vi "Arrange_FrontPanel_Object.vi"(0 "vi refnum":refnum<vi>, 7 "spacing":i32=15, 11 "error in (no error)":errorcluster) -> (4 "vi refnum out":refnum<vi>, 15 "error out":errorcluster)   [LabVIEW 2017]
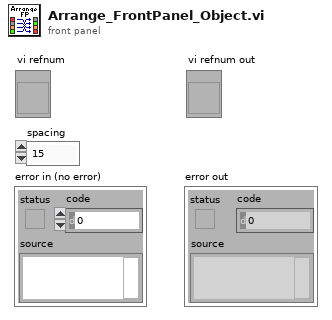
[diagram p1: front panel]
types:
  T1 = cluster{"Ctl Refnum":refnum<vi>, "width":i32, "height":i32, "label":string}
  T2 = cluster{"Ctl Refnum":refnum<vi>, "width":i32, "height":i32, "label":string}[]
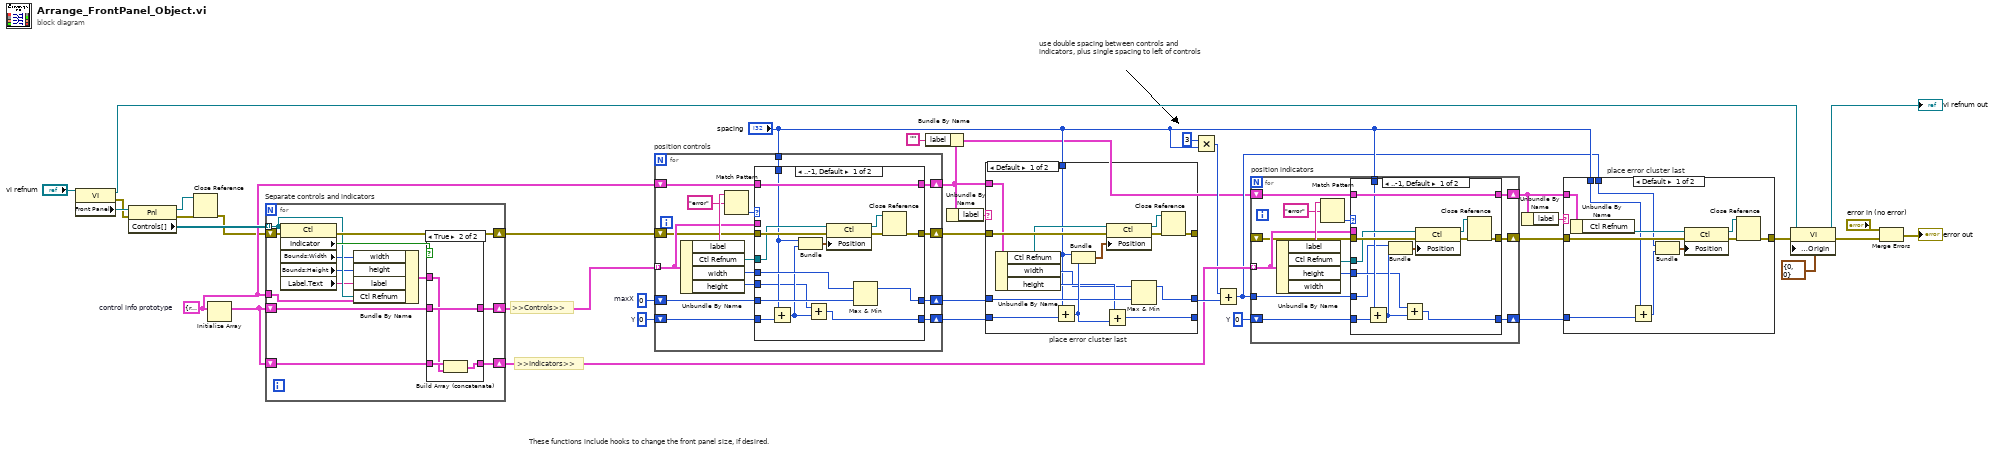
[diagram p0: block diagram]
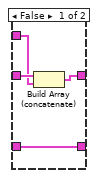
[diagram p6: hidden frame]
diagram:
  w33 = T1 {"Ctl Refnum"=refnum, "width"=0, "height"=0, "label"=""}  # control info prototype
  w18 = 0  # Y
  w29 = 0  # Y
  w31 = 0  # maxX
  # "These functions include hooks to change the front panel size, if desired."
  # "use double spacing between controls and\nindicators, plus single spacing to left of controls"
  # ">>Indicators>>"
  # ">>Controls>>"
  n1 = property class="VI"(reference="vi refnum") -> (reference out=w2:refnum<vi>, error out=w30:errorcluster, "Front Panel"=w37:refnum<vi>)  [unwired: 1 in]
  n2 = property class="Pnl"(reference=w37, error in=w30) -> (reference out=w13:refnum<vi>, error out=w14:errorcluster, "Controls[]"=w36:refnum<vi>[])
  n3 = Close Reference(reference=w13, error in (no error)=w14) -> (error out=w12:errorcluster)
  n4 = Initialize Array(w33) -> (w35:T2)  [unwired: 1 in]
  n5 = for "Separate controls and indicators" {
    shift-right: [w46] -> w32
    shift-left: w35 -> [w48]
    shift-right: [w45] -> w17
    shift-left: w35 -> [w47]
    tunnel: w36 -> [w43] mode=indexing
    shift-right: [w50] -> w34
    shift-left: w12 -> [w51]
    tunnel: w33 -> [w44]
    n6 = property class="Ctl"(reference=w43, error in=w51) -> (error out=w50:errorcluster, "Indicator"=w49:bool, "Bounds:Width"=w40:u32, "Bounds:Height"=w39:u32, "Label.Text"=w42:string)  [unwired: 1 out]
    n7 = Bundle By Name(cluster=w44, "width"=w40, "height"=w39, "label"=w42, "Ctl Refnum"=w43) -> (w41:T1)
    n8 = case shown="True" w49 {
      tunnel: w41 -> [w52 w56]
      tunnel: w48 -> [w55 w59]
      tunnel: w47 -> [w53 w58]
      tunnel: [w54 w59] -> w46
      tunnel: [w53 w57] -> w45
      frame False {
        n9 = Build Array (concatenate)(w55, w52) -> (w54:T2)
      }
      frame True {
        n10 = Build Array (concatenate)(w58, w56) -> (w57:T2)
      }
    }
  }
  n11 = for "position controls" {
    shift-right: [w66] -> w26
    shift-left: w34 -> [w67]
    shift-right: [w69] -> w8
    shift-left: w33 -> [w71]
    tunnel: w32 -> [w68] mode=indexing
    shift-right: [w72] -> w25
    shift-left: w31 -> [w73]
    shift-right: [w64] -> w24
    shift-left: w29 -> [w65]
    tunnel: "spacing" -> [w60]
    n12 = Unbundle By Name(w68) -> ("label"=w75:string, "Ctl Refnum"=w61:refnum<vi>, "width"=w63:i32, "height"=w62:i32)
    n13 = Match Pattern(string=w75, regular expression="error") -> (offset past match=w70:i32)  [unwired: 1 in, 3 out]
    n14 = case shown="..-1, Default" w70 {
      tunnel: w73 -> [w87 w94]
      tunnel: [w85 w94] -> w72
      tunnel: w71 -> [w90 _]
      tunnel: [w90 w93] -> w69
      tunnel: w68 -> [_ w93]
      tunnel: w67 -> [w89 w92]
      tunnel: [w79 w92] -> w66
      tunnel: w65 -> [w84 w91]
      tunnel: [w80 w91] -> w64
      tunnel: w63 -> [w86 _]
      tunnel: w62 -> [w81 _]
      tunnel: w61 -> [w88 _]
      tunnel: w60 -> [w83 _]
      frame ..-1, Default {
        n15 = Add(x=w83, y=w84) -> (x+y=w82:i32)
        n16 = Bundle("spacing"=w83, w82) -> (w76:cluster{"spacing":i32, i32})  [unwired: 1 in]
        n17 = Add(x=w81, y=w82) -> (x+y=w80:i32)
        n18 = property class="Ctl"(reference=w88, error in=w89, "Position"=w76) -> (reference out=w77:refnum<vi>, error out=w78:errorcluster)
        n19 = Max & Min(x=w86, y=w87) -> (max(x,y)=w85:i32)  [unwired: 1 out]
        n20 = Close Reference(reference=w77, error in (no error)=w78) -> (error out=w79:errorcluster)
      }
      frame 0.. {
        # "error cluster, save it for last"
      }
    }
  }
  n21 = Bundle By Name(cluster=w8, "label"="") -> (w7:T1)
  n22 = Unbundle By Name(w8) -> ("label"=w27:string)
  n23 = case "place error cluster last" shown="Default" w27 {
    tunnel: w8 -> [w105 _]
    tunnel: w26 -> [w106 w110]
    tunnel: w25 -> [w107 w112]
    tunnel: w24 -> [w108 w111]
    tunnel: [w100 w112] -> w23
    tunnel: [w96 w111] -> _
    tunnel: [w99 w110] -> _
    tunnel: "spacing" -> [w101 _]
    frame Default {
      n24 = Unbundle By Name(w105) -> ("Ctl Refnum"=w104:refnum<vi>, "width"=w102:i32, "height"=w103:i32)
      n25 = Add(x=w101, y=w108) -> (x+y=w109:i32)
      n26 = Bundle("spacing"=w101, w109) -> (w95:cluster{"spacing":i32, i32})  [unwired: 1 in]
      n27 = Add(x=w103, y=w109) -> (x+y=w96:i32)
      n28 = property class="Ctl"(reference=w104, error in=w106, "Position"=w95) -> (reference out=w97:refnum<vi>, error out=w98:errorcluster)
      n29 = Max & Min(x=w102, y=w107) -> (max(x,y)=w100:i32)  [unwired: 1 out]
      n30 = Close Reference(reference=w97, error in (no error)=w98) -> (error out=w99:errorcluster)
    }
    frame "" {
      # "no error cluster on\nfront panel"
    }
  }
  n31 = Multiply(x=3, y="spacing") -> (x*y=w16:i32)
  n32 = Add(x=w16, y=w23) -> (x+y=w11:i32)
  n33 = for "position indicators" {
    shift-right: [w119] -> w21
    shift-left: _ -> [w120]
    shift-right: [w122] -> w19
    shift-left: w7 -> [w124]
    tunnel: w17 -> [w121] mode=indexing
    shift-right: [w113] -> w22
    shift-left: w18 -> [w118]
    tunnel: "spacing" -> [w115]
    tunnel: w11 -> [w114]
    n34 = Unbundle By Name(w121) -> ("label"=w126:string, "Ctl Refnum"=w116:refnum<vi>, "height"=w117:i32)  [unwired: 1 out]
    n35 = Match Pattern(string=w126, regular expression="error") -> (offset past match=w123:i32)  [unwired: 1 in, 3 out]
    n36 = case shown="..-1, Default" w123 {
      tunnel: w114 -> [w131 _]
      tunnel: w124 -> [w139 _]
      tunnel: [w139 w142] -> w122
      tunnel: w121 -> [_ w142]
      tunnel: w120 -> [w138 w141]
      tunnel: [w128 w141] -> w119
      tunnel: w118 -> [w136 w140]
      tunnel: [w132 w140] -> w113
      tunnel: w117 -> [w133 _]
      tunnel: w116 -> [w137 _]
      tunnel: w115 -> [w135 _]
      frame ..-1, Default {
        n37 = Add(x=w135, y=w136) -> (x+y=w134:i32)
        n38 = Bundle(w131, w134) -> (w127:cluster{i32, i32})  [unwired: 1 in]
        n39 = Add(x=w133, y=w134) -> (x+y=w132:i32)
        n40 = property class="Ctl"(reference=w137, error in=w138, "Position"=w127) -> (reference out=w129:refnum<vi>, error out=w130:errorcluster)
        n41 = Close Reference(reference=w129, error in (no error)=w130) -> (error out=w128:errorcluster)
      }
      frame 0.. {
        # "error cluster, save it for last"
      }
    }
  }
  n42 = Unbundle By Name(w19) -> ("label"=w20:string)
  n43 = case "place error cluster last" shown="Default" w20 {
    tunnel: w19 -> [w151 _]
    tunnel: w21 -> [w152 w154]
    tunnel: w22 -> [w153 _]
    tunnel: [w147 w154] -> w5
    tunnel: "spacing" -> [w149 _]
    tunnel: w11 -> [w144 _]
    frame Default {
      n44 = Unbundle By Name(w151) -> ("Ctl Refnum"=w150:refnum<vi>)
      n45 = Add(x=w149, y=w153) -> (x+y=w148:i32)
      n46 = Bundle(w144, w148) -> (w143:cluster{i32, i32})  [unwired: 1 in]
      n47 = property class="Ctl"(reference=w150, error in=w152, "Position"=w143) -> (reference out=w145:refnum<vi>, error out=w146:errorcluster)
      n48 = Close Reference(reference=w145, error in (no error)=w146) -> (error out=w147:errorcluster)
    }
    frame "" {
      # "no error cluster on\nfront panel"
    }
  }
  n49 = property class="VI"(reference=w2, error in=w5, "Front Panel Window:Origin"=cluster{"Horizontal":i16, "Vertical":i16} {"Horizontal"=0, "Vertical"=0}) -> (reference out=→"vi refnum out":refnum<vi>, error out=w4:errorcluster)
  n50 = Merge Errors("error in (no error)", w4) -> (→"error out":errorcluster)
